vi "execute_python_function.vi"() -> ()   [LabVIEW 2021]
panel:
  out "return value":cluster{i32, string}
  out "error out":errorcluster
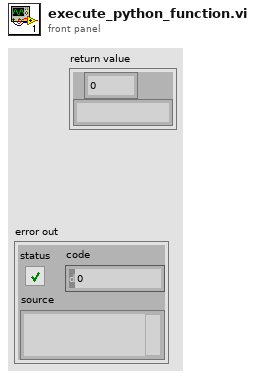
[diagram p1: front panel]
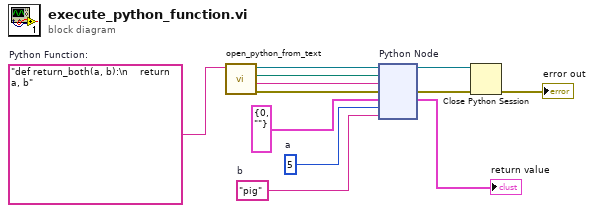
[diagram p0: block diagram]
diagram:
  w2 = 5  # a
  w4 = "pig"  # b
  w7 = "def return_both(a, b):\n    return a, b"  # Python Function:
  n1 = call "open_python_from_text.vi"("Python Function:"=w7) -> ("error out"=w10:errorcluster, "function name"=w5:string, "module path"=w6:path, "Refnum out"=w12:refnum<k35>)  [unwired: 7 in]
  n2 = node "Python Node"(w12, w6, w5, w10, cluster{i32, string} {0, ""}, w2, w4) -> (w11:refnum<k35>, w9:errorcluster, →"return value":cluster{i32, string})  [unwired: 2 in, 2 out]
  n3 = Close Python Session(session in=w11, error in=w9) -> (11:→"error out":errorcluster)
